vi "MotionProfiling_2D_NopeExample.vi"(6 "TalonPidgeonIsConnectedTo":string="DUT", 7 "PidgeonGyroName":string="DUT", 8 "error in (no error)":errorcluster, 9 "LeftMotorName":string="DUT", 10 "RightMotorName":string="DUT", 11 "file path (dialog if empty)":path=path "/home/lvuser/mp3.csv") -> (0 "error out":errorcluster)   [LabVIEW 2017]
panel:
  out "Heading":dbl(graph)
  out "Position":i32(graph)
  out "Velocity":i32(graph)
  out "Loop Time":u32(knob) scale=0.0..20.0
  # "This is an untested attempt at following a previosly-generated motion profile.  It is spliced from examples provided by CTRE, specifically the \"RemoteClosedLoop\" one. As such, it relies on the  \"ConfigureRobot\" and \"Zero Sensors\" vis as well as the \"Constants\" global variable."
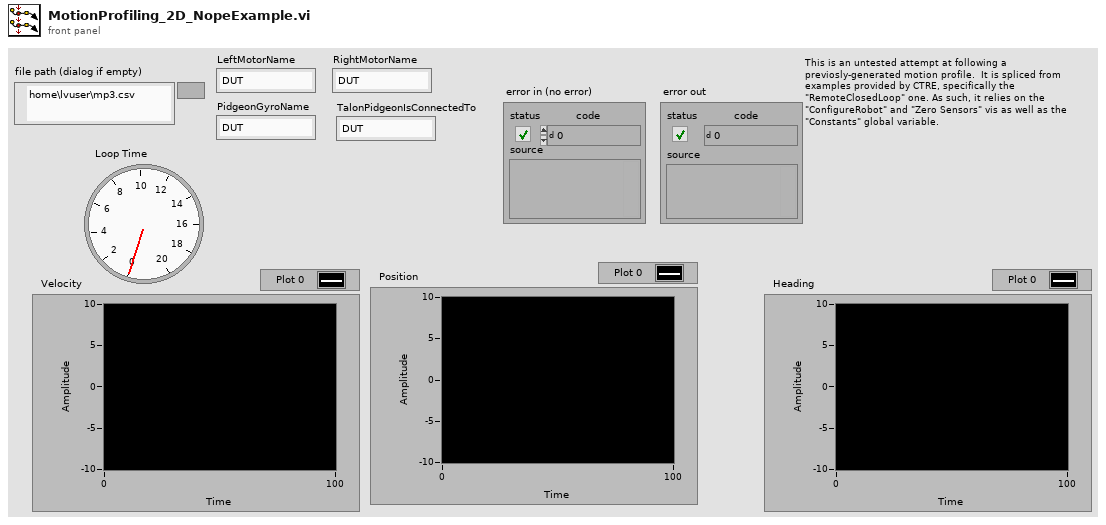
[diagram p1: front panel]
types:
  T1 = typedef "WPI_MotorControlDeviceRef.ctl" = cluster{"DeviceStatus":errorcluster, "Type":T2, "PWM":cluster{"PWM Channel":T3, "DeadBand":T4}, "CAN":cluster{"Device Number":u8, "SetOutput VI Ref":variant, "GetOutput VI Ref":variant, "Enable VI Ref":variant, "Disable VI Ref":variant, "Data":variant}, "Invert":bool, "DIO PWM":cluster{"PWM \"Enable\" Channel":T3, "DIOChannel":T5, "PWM Rate":dbl}}
  T2 = typedef "WPI_MotorControlType.ctl" = enum16{"PWM", "CAN", "DIO PWM"}
  T3 = typedef "FPGA_DIOPWMChannel.ctl" = enum8{"PWM 0", "PWM 1", "PWM 2", "PWM 3", "PWM 4", "PWM 5", "PWM 6", "PWM 7", "PWM 8", "PWM 9", "PWM MXP 0", "PWM MXP 1", "PWM MXP 2", "PWM MXP 3", "PWM MXP 4", "PWM MXP 5", "PWM MXP 6", "PWM MXP 7", "PWM MXP 8", "PWM MXP 9", "Invalid"}
  T4 = typedef "WPI_PWMDeadband.ctl" = cluster{"Name":string, "maxPositivePwm":i32, "minPositivePwm":i32, "centerPwm":i32, "maxNegativePwm":i32, "minNegativePwm":i32, "angularRange":u16}
  T5 = typedef "FPGA_DIOChannel.ctl" = enum8{"DIO 0", "DIO 1", "DIO 2", "DIO 3", "DIO 4", "DIO 5", "DIO 6", "DIO 7", "DIO 8", "DIO 9", "DIO MXP 0", "DIO MXP 1", "DIO MXP 2", "DIO MXP 3", "DIO MXP 4", "DIO MXP 5", "DIO MXP 6", "DIO MXP 7", "DIO MXP 8", "DIO MXP 9", "DIO MXP 10", "DIO MXP 11", "DIO MXP 12", "DIO MXP 13", "DIO MXP 14", "DIO MXP 15", "SPI Port CS1", "SPI Port CS2", "SPI Port CS3", "SPI Port MISO", "SPI Port MOSI", "Invalid"}
  T6 = typedef "CTRE_PigeonIMU_DeviceRef.ctl" = cluster{"DeviceStatus":errorcluster, "Device Number":u8, "Type":T7, "Device ID":u32, "Handle":u64, "UsageFrame":u32, "Library Path":path}
  T7 = typedef "CTRE_PigeonIMU_ConnectionType.ctl" = u32
  T8 = cluster{"Top Buffer Remaining":i32, "Top Buffer Count":i32, "Bottom Buffer Count":i32, "Has Underrun?":bool, "Is Underrun?":bool, "Active Point Valid?":bool, "Is Last?":bool, "Profile Slot Select 0":i32, "Output Enable":i32, "Time Duration (ms)":i32, "Profile Slot Select 1":i32}
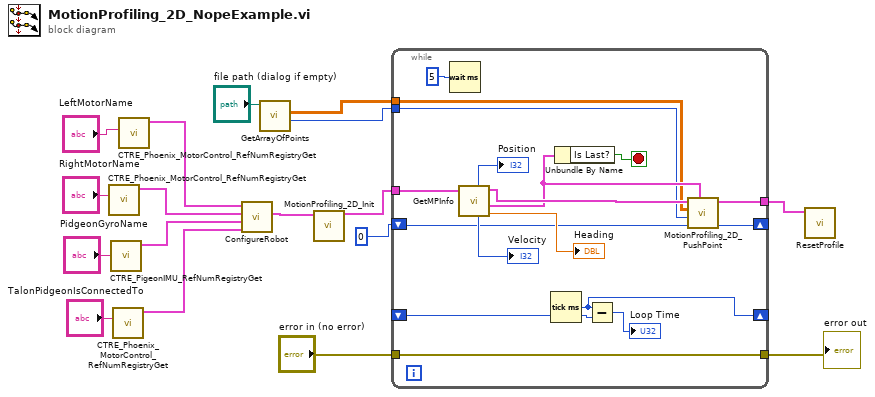
[diagram p0: block diagram]
diagram:
  n1 = call <vilib>:"CTRE_Phoenix_MotorControl_RefNumRegistryGet.vi"("refnum name"="RightMotorName") -> ("PhoenixMotorControlDevRef"=w9:T1)  [unwired: 9 in, 1 out]
  n2 = call <vilib>:"CTRE_PigeonIMU_RefNumRegistryGet.vi"("refnum name"="PidgeonGyroName") -> ("PigeonIMUDevRef"=w7:T6)  [unwired: 9 in, 1 out]
  n3 = call <vilib>:"CTRE_Phoenix_MotorControl_RefNumRegistryGet.vi"("refnum name"="TalonPidgeonIsConnectedTo") -> ("PhoenixMotorControlDevRef"=w5:T1)  [unwired: 9 in, 1 out]
  n4 = call <vilib>:"CTRE_Phoenix_MotorControl_RefNumRegistryGet.vi"("refnum name"="LeftMotorName") -> ("PhoenixMotorControlDevRef"=w11:T1)  [unwired: 9 in, 1 out]
  n5 = call "ConfigureRobot.vi"("Pigeon Talon"=w5, "Pigeon"=w7, "Right Side"=w9, "Left Side"=w11) -> ("Right Side"=w2:T1)  [unwired: 5 in, 2 out]
  n6 = call "GetArrayOfPoints.vi"("file path (dialog if empty)"="file path (dialog if empty)") -> ("Number of Points"=w15:i32, "Array of Trajectory Points"=w16:dbl[][])  [unwired: 9 in]
  n7 = call "MotionProfiling_2D_Init.vi"("RightTalon"=w2) -> ("RightTalonOut"=w1:T1)  [unwired: 10 in]
  n8 = while {
    tunnel: w1 -> [w22]
    shift-right: [w25] -> _
    shift-left: u32 0 ("milliseconds to wait") -> [w24]
    tunnel: w16 -> [w19]
    tunnel: w15 -> [w18]
    tunnel: [w30] -> w14
    tunnel: "error in (no error)" -> [w30]
    shift-right: [w29] -> _
    shift-left: _ -> [w28]
    tunnel: [w21] -> w3
    stop <- w31 stop-if-true
    n9 = Wait (ms)(milliseconds to wait=u32 5) -> ()  [unwired: 1 out]
    n10 = call "GetMPInfo.vi"("PhoenixMotorControlDevRef"=w22) -> ("Heading"=→"Heading":dbl, "Motion Profile Status"=w20:T8, "PhoenixMotorControlDevRef Out"=w23:T1, "Velocity (Sensor Units per 100 ms)"=→"Velocity":i32, "Position (Sensor Units)"=→"Position":i32)  [unwired: 5 in, 1 out]
    n11 = Tick Count (ms)() -> (millisecond timer value=w29:u32)
    n12 = Unbundle By Name(w20) -> ("Is Last?"=w31:bool)
    n13 = Subtract(x=w29, y=w28) -> (x-y=→"Loop Time":u32)
    n14 = call "MotionProfiling_2D_PushPoint.vi"("Motion Profile Status"=w20, "CursorIn"=w24, "NumberOfPoints"=w18, "ArrayOfTrajectoyPoints"=w19, "PhoenixMotorControlDevRef"=w23) -> ("CursorOut"=w25:u32, "PhoenixMotorControlDevRef Out"=w21:T1)  [unwired: 5 in]
  }
  "error out" <- w14
  n15 = call "ResetProfile.vi"("PhoenixMotorControlDevRef"=w3) -> ()  [unwired: 10 in, 1 out]
